vi "C37 Get PDC Data.vi"(8 "error in (no error)":errorcluster, 11 "Pseudo PDC ID":i32) -> (0 "error out":errorcluster, 3 "PDC Data":T1)   [LabVIEW 2013, in "C37118-DLL.lvlib"]
uses:
  C37118-DLL.lvlib
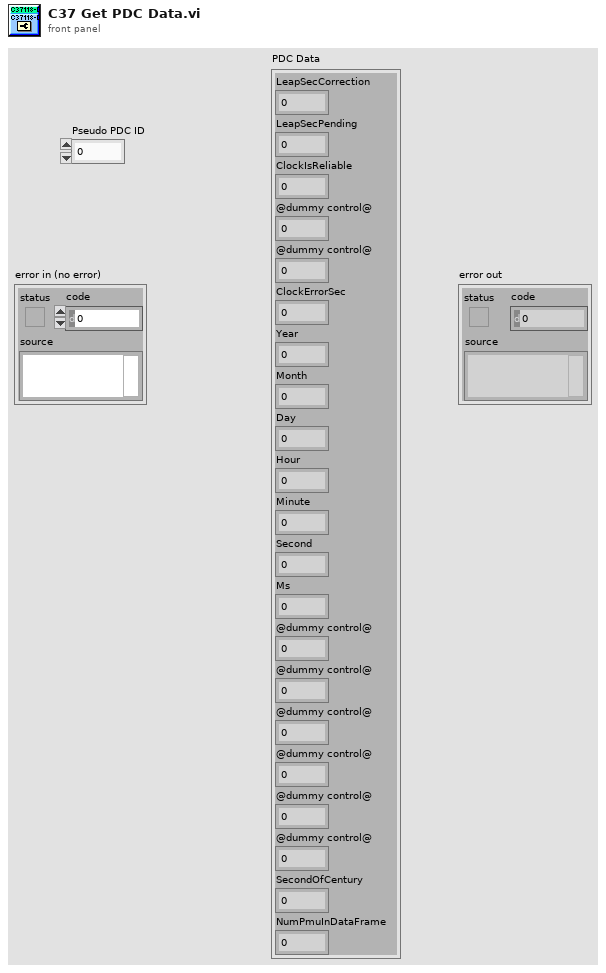
[diagram p1: front panel]
types:
  T1 = cluster{"LeapSecCorrection":i32, "LeapSecPending":u8, "ClockIsReliable":u8, "@dummy control@":i8, "@dummy control@":i8, "ClockErrorSec":sgl, "Year":i16, "Month":i16, "Day":i16, "Hour":i16, "Minute":i16, "Second":i16, "Ms":i16, "@dummy control@":i8, "@dummy control@":i8, "@dummy control@":i8, "@dummy control@":i8, "@dummy control@":i8, "@dummy control@":i8, "SecondOfCentury":dbl, "NumPmuInDataFrame":i32}
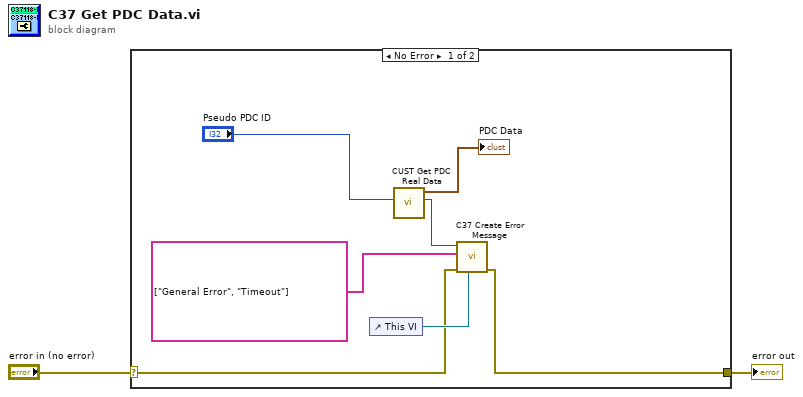
[diagram p0: block diagram]
diagram:
  n1 = case shown="No Error" "error in (no error)" {
    selector: "error in (no error)" -> [w8 w10]
    tunnel: [w7 w10] -> w2
    frame No Error {
      n2 = control-ref of="This VI"() -> (w9:refnum<vi>)
      n3 = call "CUST Get PDC Real Data.vi"("pseudoPdcId"="Pseudo PDC ID") -> ("function return"=w4:i32, "rd out"=→"PDC Data":T1)  [unwired: 9 in]
      n4 = call "C37 Create Error Message.vi"("VI Reference"=w9, "error in (no error)"=w8, "Error Messages"=string[] ["General Error", "Timeout"], "function return"=w4) -> ("error out"=w7:errorcluster)  [unwired: 7 in]
    }
    frame Error {
    }
  }
  "error out" <- w2
